vi "Configure Hardware.vi"(8 "error in (no error)":errorcluster, 11 "Hardware Resources in":T1 {"Reference Distance" format="%.3g"}) -> (0 "error out":errorcluster, 3 "Hardware Resources out":T1 {"Reference Distance" format="%.3g"})   [LabVIEW 2018, in "Acquisition.lvlib"]
doc: "Configure the hardware."
uses:
  Acquisition.lvlib
  Hardware Configuration.ctl
  <vilib>/Instr/_visa.llb/VISA Configure Serial Port (Instr).vi
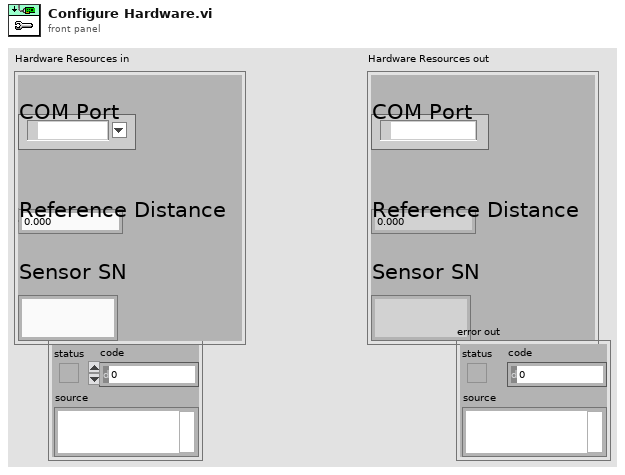
[diagram p1: front panel]
types:
  T1 = typedef "Acquisition.lvlib/Hardware Configuration.ctl" = cluster{"COM Port":refnum<visa-resource-name>, "Reference Distance":dbl, "Sensor SN":string}
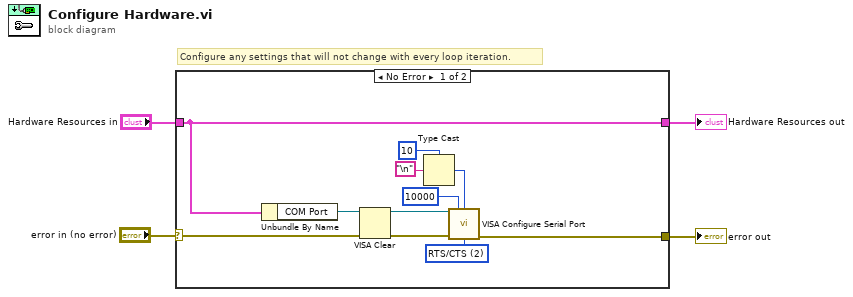
[diagram p0: block diagram]
diagram:
  # "Configure any settings that will not change with every loop iteration."
  n1 = case shown="No Error" "error in (no error)" {
    selector: "error in (no error)" -> [w8 w16]
    tunnel: [w7 w16] -> w3
    tunnel: "Hardware Resources in" -> [w15 w17]
    tunnel: [w15 w17] -> w1
    frame No Error {
      w12 = u16 2 items=["None", "XON/XOFF", "RTS/CTS", "XON/XOFF & RTS/CTS", "DTR/DSR", "XON/XOFF & DTR/DSR"] ("flow control (0:none)")
      n2 = Unbundle By Name(w15) -> ("COM Port"=w6:refnum<visa-resource-name>)
      n3 = VISA Clear(VISA resource name=w6, error in (no error)=w8) -> (VISA resource name out=w14:refnum<visa-resource-name>, error out=w13:errorcluster)
      n4 = Type Cast(type=u8 10 ("termination char\n(0xA = '\\n' = LF)"), x="\n") -> (*(type *) &x=w9:u8)
      n5 = call-poly "VISA Configure Serial Port"("VISA resource name"=w14, "timeout (10sec)"=u32 10000, "termination char\n(0xA = '\\n' = LF)"=w9, "error in (no error)"=w13, "flow control (0:none)"=w12) -> ("error out"=w7:errorcluster)  [unwired: 9 in, 1 out]
    }
    frame Error {
    }
  }
  "Hardware Resources out" <- w1
  "error out" <- w3
